vi "Create FFID Auto Calib setup file.vi"(3 "Results filename":string, 5 "Auto_Calib_Setup.xls":string="Auto_Calib_Setup.xls", 6 "Traverse line":T1 {"Carrier_2 Q (l/min)" format="%#.2f"; "Row Duration (mins)" format="%#.1f"; "Row No" min=0; "Trace Gas Concentration (%)" min=0.0 format="%#_4f"; "Carrier_1 Q (l/min)" format="%#.4f"; "Start X" format="%#.2f"; "Start Y" format="%#.2f"; "Start Z" format="%#.2f"; "End X" format="%#.2f"; "End Y" format="%#.2f"; "End Z" format="%#.2f"; "Tunnel Speed" format="%#.2f"; "Averaging time (mins)" min=0.0 format="%#.2f"}) -> (1 "HFR500 Comms Channels":string[](array[string]))   [LabVIEW 2022 SP3]
uses:
  Gen Trav/Traverse_cluster.ctl
  Gen Trav/Spacing.ctl
  Controls/Multi_run_mode.ctl
  File/Setup_Filetype.ctl
panel:
  # "X           Y          Z"
  # "Start"
  # "End"
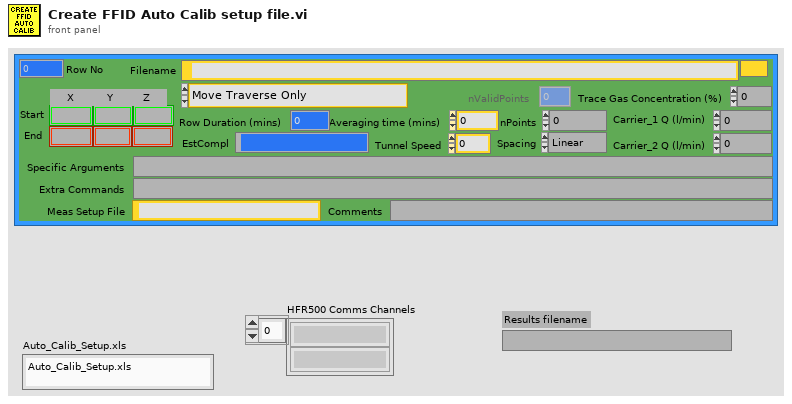
[diagram p1: front panel]
types:
  T1 = typedef "Traverse_cluster.ctl" = cluster{"Start X":sgl, "Start Y":sgl, "Start Z":sgl, "End X":sgl, "End Y":sgl, "End Z":sgl, "nPoints":i32, "Spacing":T2, "Filename":path, "Tunnel Speed":dbl, "Averaging time (mins)":dbl, "Extra Commands":string, "Carrier_1 Q (l/min)":dbl, "Carrier_2 Q (l/min)":dbl, "Trace Gas Concentration (%)":dbl, "Specific Arguments":string, "Comments":string, "Row No":i32, "Row Type Selector":T3, "EstCompl":string, "Row Duration (mins)":dbl, "nValidPoints":i32, "Meas Setup File":string}
  T2 = typedef "Spacing.ctl" = enum16{"Linear", "Log", "Gauss", "Specified", "N/A"}
  T3 = typedef "Multi_run_mode.ctl" = enum16{"Move Traverse Only", "Set Tunnel Speed Only", "Set Source Only", "Set Measurement Conditions", "Single Measurement", "Vertical Profile", "Lateral Profile", "Longitudinal Profile", "Multi-Axis Profile", "Explore Volume", "Auto Calibrate", "Meas Fast FID Bkgnd", "Check Beam Power", "Scanning Valve Measurement", "Run VI Named:", "Set ADAM Ch", "Wait (minutes)", "Send Message", "Synchronize With:", "Fall Back to this Row", "Turn Off Row Repeating", "Traverse 3D Volume", "Blank Row", "Jump to Fall Back Row"}
  T4 = typedef "Setup_Filetype.ctl" = enum16{"Measurement Setups", "Calibration Setups", "General", "Results File Plotter Setups", "Speed Calib Tweaks"}
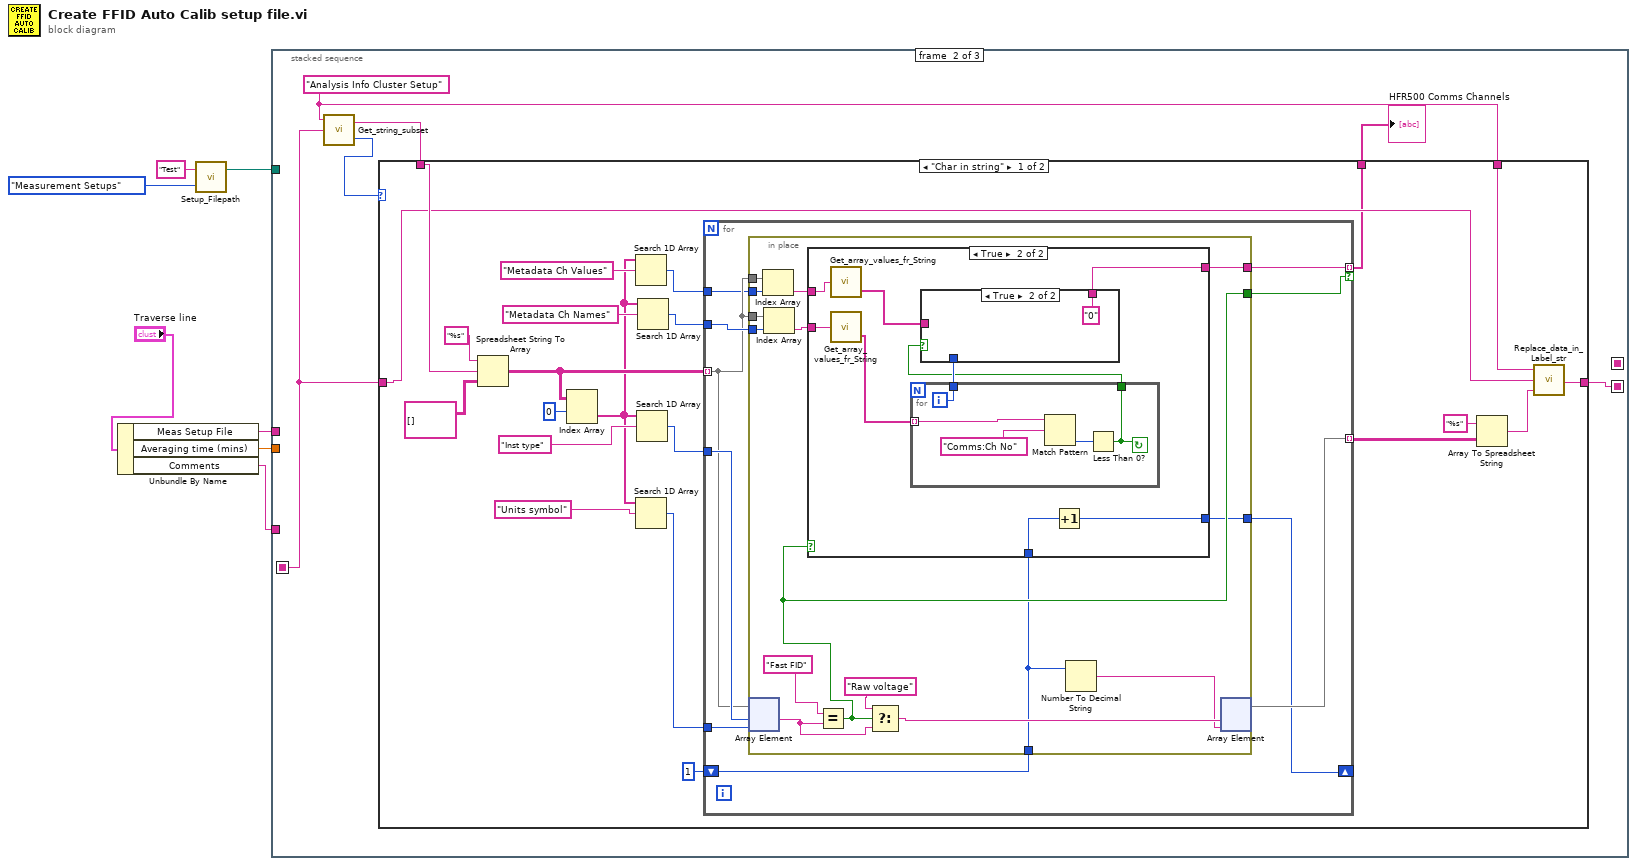
[diagram p0: block diagram]
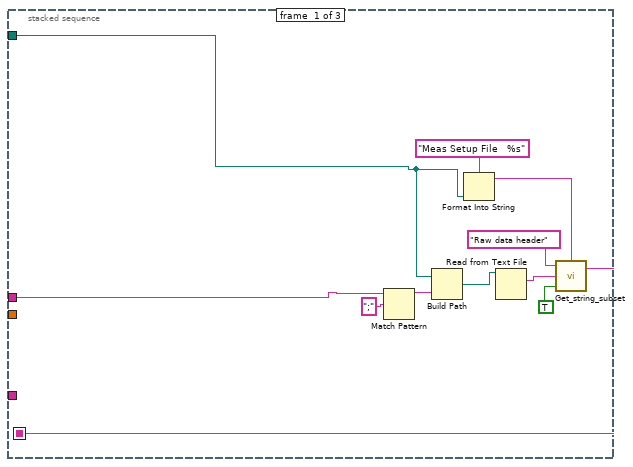
[diagram p2: hidden frame]
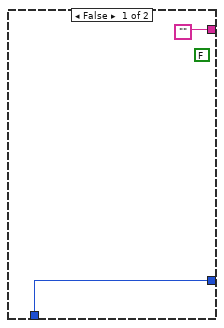
[diagram p3: hidden frame]
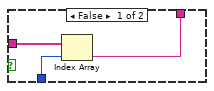
[diagram p4: hidden frame]
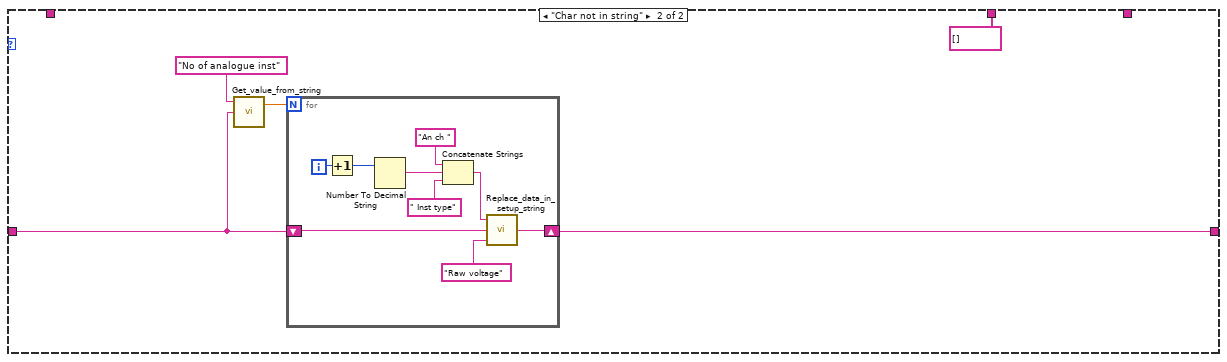
[diagram p5: hidden frame]
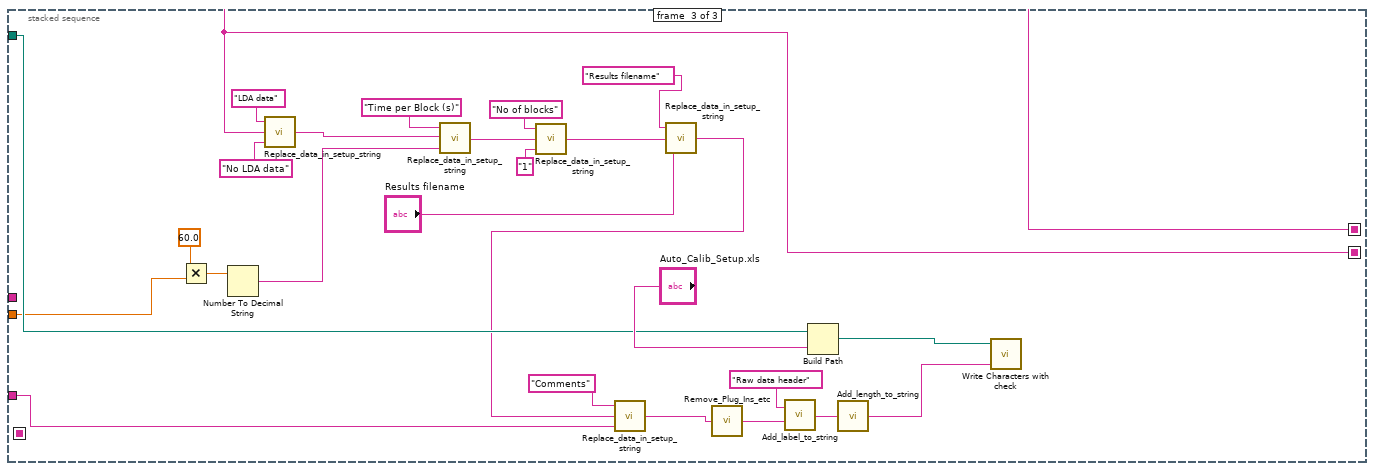
[diagram p6: hidden frame]
diagram:
  n1 = Unbundle By Name("Traverse line") -> ("Meas Setup File"=w3:string, "Averaging time (mins)"=w2:dbl, "Comments"=w1:string)
  n2 = call "Setup_Filepath.vi"("Setup File Type"=Setup_Filetype."Measurement Setups", "Filename in"="Test") -> ("Directory"=w7:path)  [unwired: 1 out]
  n3 = stacked-sequence {
    seq-local: [_ w20 _] -> [_ _ w122]
    seq-local: [_ _ w122] -> [_ _ _]
    seq-local: [w11 _ _] -> [_ w21 _]
    tunnel: w7 -> [w10 _ w116]
    tunnel: w3 -> [w8 _ _]
    tunnel: w2 -> [_ _ w110]
    tunnel: w1 -> [_ _ w106]
    frame #0 {
      n4 = Match Pattern(string=w8, regular expression=";") -> (before substring=w14:string)  [unwired: 4 out]
      n5 = Build Path(base path=w10, name or relative path=w14) -> (appended path=w9:path)
      n6 = Format Into String(format string="Meas Setup File   %s", w10) -> (resulting string=w12:string)  [unwired: 2 in, 1 out]
      n7 = Read from Text File(file (use dialog)=w9) -> (text=w17:string)  [unwired: 3 in, 3 out]
      n8 = call "Get_string_subset.vi"("String Name"=w12, "Show Dialog?"=TRUE, "String to split"=w17, "File Label"="Raw data header") -> ("Output string"=w11:string)  [unwired: 1 out]
    }
    frame #1 {
      w22 = "Analysis Info Cluster Setup"
      n9 = call "Get_string_subset.vi"("String to split"=w21, "File Label"=w22) -> ("Status"=w24:enum16{"Char in string", "Char not in string"}, "Output string"=w23:string)  [unwired: 2 in]
      n10 = case shown="\"Char in string\"" w24 {
        tunnel: [w35 w96] -> w20
        tunnel: w21 -> [w34 w93]
        tunnel: w23 -> [w42 _]
        tunnel: w22 -> [w37 _]
        tunnel: [w29 string[] []] -> w19
        frame "Char in string" {
          n11 = Spreadsheet String To Array(format string="%s", spreadsheet string=w42, array type (2D Dbl)=string[][] []) -> (array=w40:string[][])  [unwired: 1 in]
          n12 = Index Array(array=w40, index (row)=0) -> (element=w28:string[])  [unwired: 1 in]
          n13 = Search 1D Array(1D array=w28, element="Metadata Ch Values") -> (index of element=w30:i32)  [unwired: 1 out]
          n14 = Search 1D Array(1D array=w28, element="Units symbol") -> (index of element=w26:i32)  [unwired: 1 out]
          n15 = Search 1D Array(1D array=w28, element="Inst type") -> (index of element=w41:i32)  [unwired: 1 out]
          n16 = Search 1D Array(1D array=w28, element="Metadata Ch Names") -> (index of element=w32:i32)  [unwired: 1 out]
          n17 = for {
            tunnel: w41 -> [w56]
            tunnel: w40 -> [w53] mode=indexing
            tunnel: [w55] -> w38 mode=indexing
            tunnel: w32 -> [w54]
            tunnel: w30 -> [w52]
            tunnel: [w51] -> w29 mode=indexing if=w50
            tunnel: w26 -> [w49]
            shift-right: [w47] -> _
            shift-left: 1 -> [w48]
            n18 = in-place {
              in-place-border: w53 -> [w66]
              in-place-border: w54 -> [w65]
              in-place-border: w53 -> [w64]
              in-place-border: w52 -> [w63]
              in-place-border: [w60] -> w50
              in-place-border: [w61] -> w51
              in-place-border: w48 -> [w58]
              in-place-border: [w59] -> w47
              n19 = in-place-array #1 ("Array Index / Replace Elements")(w53, w56, w49) -> (w69:string)  [unwired: 1 out]
              n20 = Index Array(array=w64, index=w63) -> (element=w62:string)
              n21 = Index Array(array=w66, index=w65) -> (element=w67:string)
              n22 = Equal?(x="Fast FID", y=w69) -> (x = y?=w60:bool)
              n23 = case shown="True" w60 {
                tunnel: w67 -> [_ w82]
                tunnel: w62 -> [_ w80]
                tunnel: ["" w77] -> w61
                tunnel: w58 -> [w72 w75]
                tunnel: [w72 w74] -> w59
                frame False {
                  (unwired) FALSE
                }
                frame True {
                  n24 = call "Get_array_values_fr_String.vi"("String Value"=w80) -> ("String array"=w78:string[])  [unwired: 1 out]
                  n25 = call "Get_array_values_fr_String.vi"("String Value"=w82) -> ("String array"=w81:string[])  [unwired: 1 out]
                  n26 = for {
                    tunnel: w81 -> [w91] mode=indexing
                    tunnel: [w88] -> w79
                    tunnel: [w87] -> w76
                    i -> [w88]
                    stop <- w87 continue-if-true
                    n27 = Match Pattern(string=w91, regular expression="Comms:Ch No") -> (offset past match=w89:i32)  [unwired: 1 in, 3 out]
                    n28 = Less Than 0?(x=w89) -> (x < 0?=w87:bool)
                  }
                  n29 = case shown="True" w76 {
                    tunnel: w79 -> [w85 _]
                    tunnel: w78 -> [w84 _]
                    tunnel: [w83 "0"] -> w77
                    frame False {
                      n30 = Index Array(array=w84, index=w85) -> (element=w83:string)
                    }
                    frame True {
                    }
                  }
                  n31 = Increment(x=w75) -> (x+1=w74:i32)
                }
              }
              n32 = Select(t="Raw voltage", s=w60, f=w69) -> (s? t:f=w68:string)
              n33 = Number To Decimal String(number=w58) -> (decimal integer string=w57:string)  [unwired: 1 in]
              n34 = in-place-array #1(w68, w57) -> (w55:string[])  [unwired: 2 out]
            }
          }
          n35 = Array To Spreadsheet String(array=w38, 3:"%s" ("format string")) -> (spreadsheet string=w36:string)  [unwired: 1 in]
          n36 = call "Replace_data_in_Label_str.vi"("New data string"=w36, "Input string"=w34, "Variable name"=w37) -> ("Appended string"=w35:string)
        }
        frame "Char not in string" {
          n37 = call "Get_value_from_string.vi"("Input string"=w93, "Variable name"="No of analogue inst") -> ("Value"=w94:dbl)  [unwired: 1 in, 1 out]
          n38 = for {
            N: w94 -> [_]
            shift-right: [w97] -> w96
            shift-left: w93 -> [w99]
            i -> [w103]
            n39 = Increment(x=w103) -> (x+1=w102:i32)
            n40 = Number To Decimal String(number=w102) -> (decimal integer string=w105:string)  [unwired: 1 out]
            n41 = Concatenate Strings("An ch ", w105, " Inst type") -> (w100:string)
            n42 = call "Replace_data_in_setup_string.vi"("New data string"="Raw voltage", "Input string"=w99, "Variable name"=w100) -> ("Appended string"=w97:string)
          }
        }
      }
      "HFR500 Comms Channels" <- w19
    }
    frame #2 {
      n43 = Multiply(x=60.0, y=w110) -> (x*y=w131:dbl)
      n44 = Number To Decimal String(number=w131) -> (decimal integer string=w129:string)  [unwired: 1 out]
      n45 = call "Replace_data_in_setup_string.vi"("New data string"="No LDA data", "Input string"=w122, "Variable name"="LDA data" ("Label for characters")) -> ("Appended string"=w121:string)
      n46 = call "Replace_data_in_setup_string.vi"("New data string"=w129, "Input string"=w121, "Variable name"="Time per Block (s)") -> ("Appended string"=w128:string)
      n47 = call "Replace_data_in_setup_string.vi"("New data string"="1" ("Value"), "Input string"=w128, "Variable name"="No of blocks") -> ("Appended string"=w112:string)
      n48 = call "Replace_data_in_setup_string.vi"("New data string"="Results filename", "Input string"=w112, "Variable name"="Results filename") -> ("Appended string"=w109:string)
      n49 = call "Replace_data_in_setup_string.vi"("New data string"=w106, "Input string"=w109, "Variable name"="Comments") -> ("Appended string"=w108:string)
      n50 = call "Remove_Plug_Ins_etc.vi"("Input String"=w108) -> ("Output string"=w119:string)
      n51 = call "Add_label_to_string.vi"("String to write"=w119, "File Label"="Raw data header") -> ("Output string"=w120:string)
      n52 = Build Path(base path=w116, name or relative path="Auto_Calib_Setup.xls") -> (appended path=w115:path)
      n53 = call "Add_length_to_string.vi"("String in"=w120) -> ("String out"=w114:string)
      n54 = call "Write Characters with check.vi"("String to Write"=w114, "file (use dialog)"=w115) -> ()  [unwired: 2 in, 1 out]
    }
  }
